vi "Agilent SNA Read External Trigger Mode.vi"(7 "Agilent SNA":T1, 8 "error in (no error)":errorcluster, 11 "VISA Resource Names":T3) -> (0 "error out":errorcluster, 2 "Ext. Trigger Mode":T2, 3 "dup VISA Resource Names":T3)   [LabVIEW 2011]
doc: "This VI for the HP8753B Network Analyzers reads the stimulus values. Except when performing log sweeps and freq list sweeps, this VI uses the start and stop values and the number of points to calcuate the stimulus values."
uses:
  TypeDefs/Agilent SNA External Trigger Mode.ctl
  TypeDefs/Agilent SNA Instrument Info.ctl
  TypeDefs/Agilent SNA VISA.ctl
panel:
  in  "Channel":i8=1 min=1 max=99 step=1
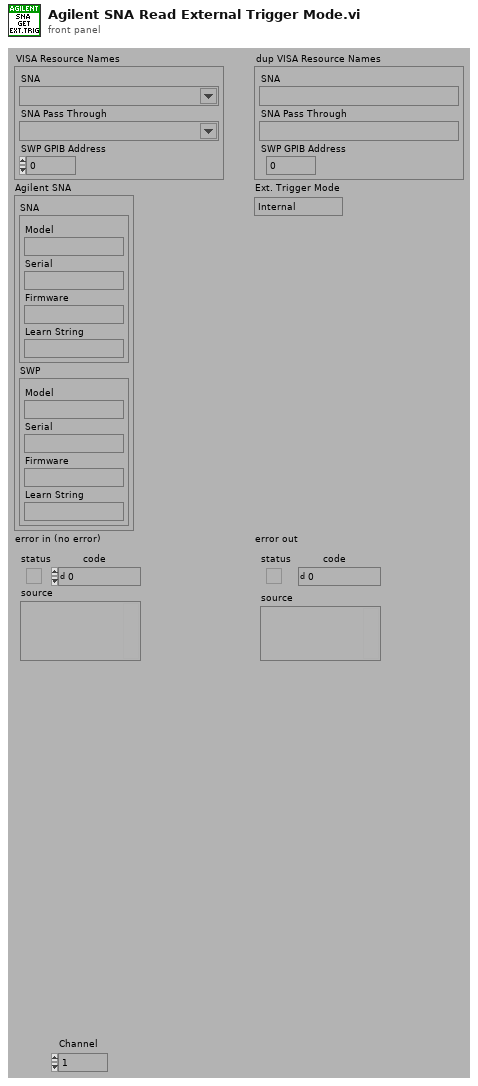
[diagram p1: front panel]
types:
  T1 = typedef "Agilent SNA Instrument Info.ctl" = cluster{"SNA":cluster{"Model":string, "Serial":string, "Firmware":string, "Learn String":string}, "SWP":cluster{"Model":string, "Serial":string, "Firmware":string, "Learn String":string}}
  T2 = typedef "Agilent SNA External Trigger Mode.ctl" = enum16{"Internal", "External", "Single/Bus"}
  T3 = typedef "Agilent SNA VISA.ctl" = cluster{"SNA":refnum<visa-resource-name>, "SNA Pass Through":refnum<visa-resource-name>, "SWP GPIB Address":i32}
  T4 = typedef "Agilent SNA Model.ctl" = enum16{"Not Supported", "8757X"}
  T5 = typedef "Agilent SNA SWP Model.ctl" = enum16{"Not Supported", "836XXX", "8375XX", "E82X7D"}
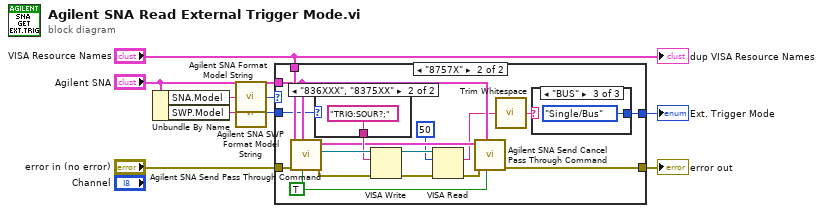
[diagram p0: block diagram]
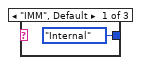
[diagram p3: hidden frame]
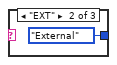
[diagram p4: hidden frame]
diagram:
  n1 = Unbundle By Name("Agilent SNA") -> ("SNA.Model"=w9:string, "SWP.Model"=w7:string)
  n2 = call "Agilent SNA Format Model String.vi"("Model String"=w9) -> ("Model"=w8:T4)
  n3 = call "Agilent SNA SWP Format Model String.vi"("Model String"=w7) -> ("Model"=w6:T5)
  n4 = case shown="\"8757X\"" w8 {
    tunnel: "VISA Resource Names" -> [_ w26]
    tunnel: "error in (no error)" -> [w10 w27]
    tunnel: [w10 w22] -> w3
    tunnel: "Agilent SNA" -> [_ w20]
    tunnel: w6 -> [_ w19]
    tunnel: [_ w13] -> w1
    frame "Not Supported" {
    }
    frame "8757X" {
      w11 = TRUE ("SCPI? (F)")
      n5 = call "Agilent SNA Send Pass Through Command.vi"("SCPI? (F)"=w11, "Agilent SNA & SWP"=w20, "error in (no error)"=w27, "VISA Resource Names"=w26) -> ("error out"=w23:errorcluster, "SNA Pass Through"=w25:refnum<visa-resource-name>, "dup VISA Resource Names"=w21:T3)  [unwired: 5 in]
      n6 = case shown="\"836XXX\", \"8375XX\"" w19 {
        tunnel: [_ "TRIG:SOUR?;"] -> w24
        frame "Not Supported" {
        }
        frame "836XXX", "8375XX" {
        }
      }
      n7 = VISA Write(VISA resource name=w25, write buffer=w24, error in (no error)=w23) -> (VISA resource name out=w17:refnum<visa-resource-name>, error out=w18:errorcluster)  [unwired: 1 out]
      n8 = VISA Read(VISA resource name=w17, byte count=u32 50, error in (no error)=w18) -> (read buffer=w14:string, error out=w16:errorcluster)  [unwired: 2 out]
      n9 = call "Agilent SNA Send Cancel Pass Through Command.vi"("SCPI? (F)"=w11, "Agilent SNA & SWP"=w20, "error in (no error)"=w16, "VISA Resource Names"=w21) -> ("error out"=w22:errorcluster)  [unwired: 6 in, 1 out]
      n10 = call <vilib>:"Trim Whitespace.vi"("string"=w14) -> ("trimmed string"=w12:string)  [unwired: 1 in]
      n11 = case shown="\"BUS\"" w12 {
        tunnel: [Agilent_SNA_External_Trigger_Mode."Internal" Agilent_SNA_External_Trigger_Mode."External" Agilent_SNA_External_Trigger_Mode."Single/Bus"] -> w13
        frame "IMM", Default {
        }
        frame "EXT" {
        }
        frame "BUS" {
        }
      }
    }
  }
  "error out" <- w3
  "Ext. Trigger Mode" <- w1
  "dup VISA Resource Names" <- "VISA Resource Names"
